vi "Read device_handle.vi"(8 "error in (no error)":errorcluster, 11 "Dali_usb_tridonics in":refnum<class "Dali_usb_tridonics.lvclass">) -> (0 "error out":errorcluster, 2 "device_handle":i32, 3 "Dali_usb_tridonics out":refnum<class "Dali_usb_tridonics.lvclass">)   [LabVIEW 2014, in "Driver_interaction.lvlib" / "Dali_usb_tridonics.lvclass"]
uses:
  Dali_usb_tridonics.lvclass
  Dali_usb_tridonics.lvclass/Dali_usb_tridonics.ctl
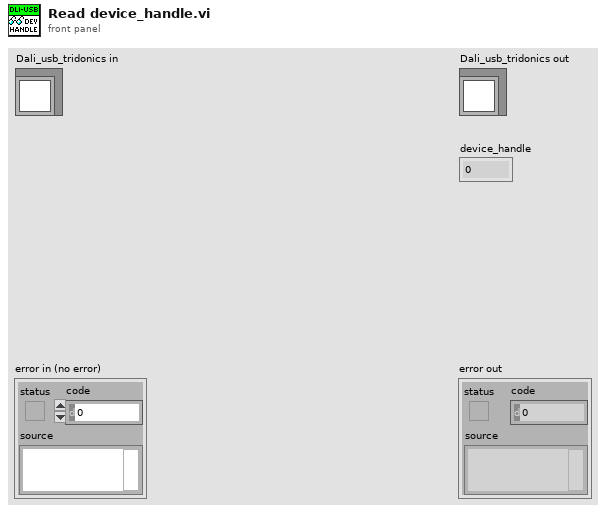
[diagram p1: front panel]
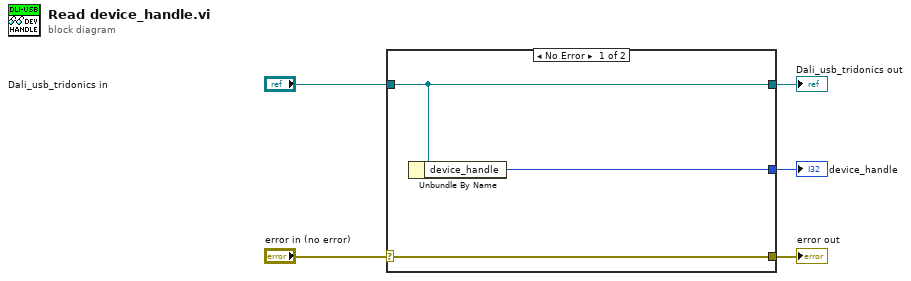
[diagram p0: block diagram]
diagram:
  n1 = case shown="No Error" "error in (no error)" {
    selector: "error in (no error)" -> [w8 w9]
    tunnel: [w8 w9] -> w4
    tunnel: [w7 w10] -> w2
    tunnel: "Dali_usb_tridonics in" -> [w7 w10]
    tunnel: [w6 _] -> w1
    frame No Error {
      n2 = Unbundle By Name(w7) -> ("device_handle"=w6:i32)
    }
    frame Error {
    }
  }
  "error out" <- w4
  "Dali_usb_tridonics out" <- w2
  "device_handle" <- w1
